vi "ST5520_TEST.vi"(8 "errin":errorcluster, 9 "key":string, 10 "lbl log std":string, 11 "ST5520":refnum<visa-resource-name>) -> (0 "errout":errorcluster, 2 "LOG STD":string, 3 "OK?":bool)   [LabVIEW 2020]
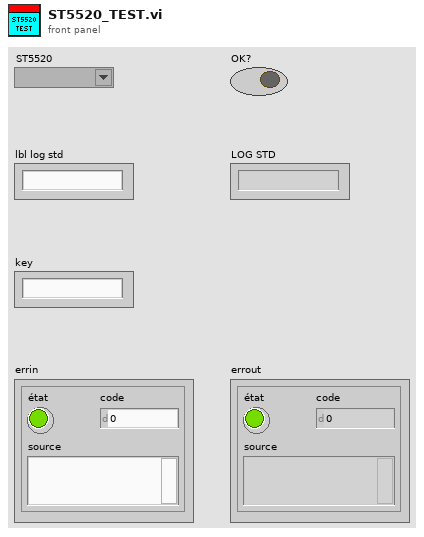
[diagram p1: front panel]
types:
  T1 = enum16{"Normal", "Over Flow", "Under Flow", "Error"}
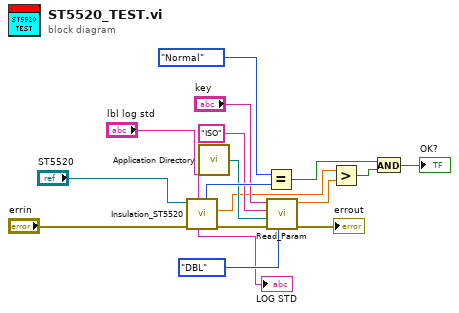
[diagram p0: block diagram]
diagram:
  n1 = call <userlib>:"Insulation_ST5520.vi"("lbl log std"="lbl log std", "errin"="errin", "Refnum VISA en entrée"="ST5520") -> ("error out"=w12:errorcluster, "R iso(MOhm)"=w3:dbl, "Status"=w13:T1, "LOG STD"=→"LOG STD":string)  [unwired: 5 out]
  n2 = call <vilib>:"Application Directory.vi"() -> ("Application Directory"=w4:path)
  n3 = Equal?(x=T1."Normal" ("Status"), y=w13) -> (x = y?=w16:bool)
  n4 = call <userlib>:"Read_Param.vi"("Énum"=enum16{"STR", "DBL", "U32"}."DBL", "errin"=w12, "pathin"=w4, "section"="ISO", "key"="key") -> ("error out"=→"errout":errorcluster, "dbl"=w8:dbl)  [unwired: 2 in, 3 out]
  n5 = Greater?(x=w3, y=w8) -> (0:w15:bool)
  n6 = And(x=w16, y=w15) -> (x .and. y?=→"OK?":bool)
